vi "MU Load Register.vi"(7 "count in":u32, 8 "error in (no error)":errorcluster, 9 "address":u32, 10 "filepath":string, 11 "handle":u64) -> (0 "error out (no error)":errorcluster, 1 "count out":u32, 2 "values":u32[](array[numeric]), 3 "function return":u32)   [LabVIEW 2017, in "MU_3SL_interface.lvlib"]
uses:
  MU_3SL_interface.lvlib
  lib/MU_3SL_interface.dll
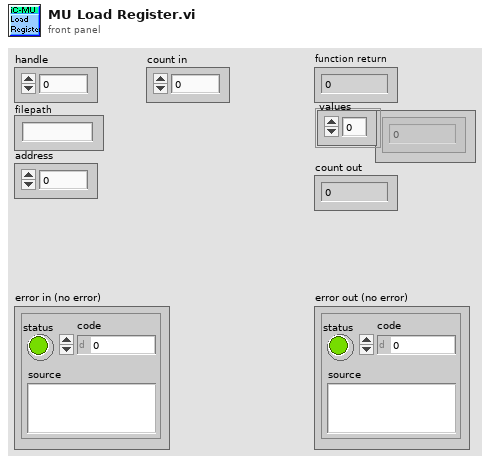
[diagram p1: front panel]
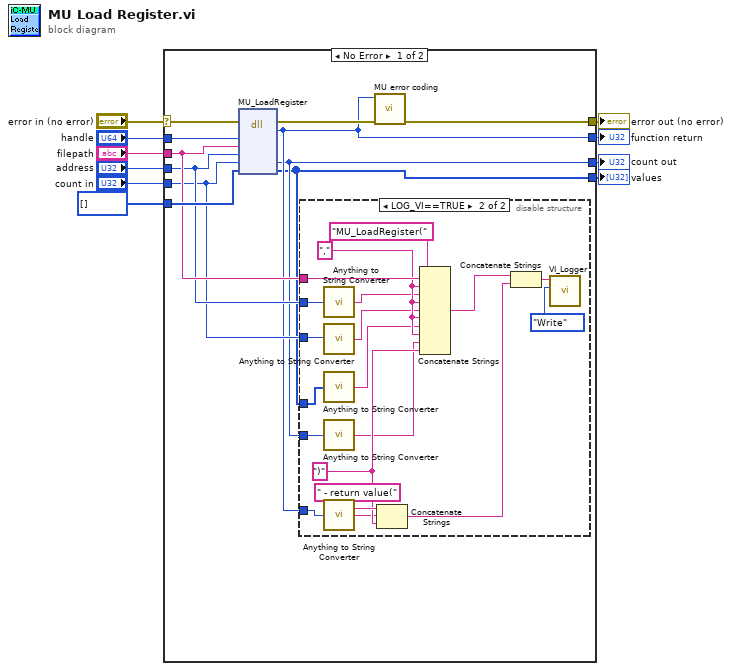
[diagram p0: block diagram]
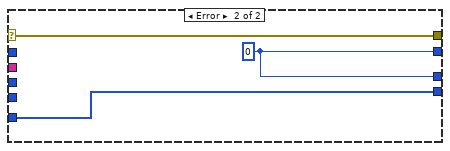
[diagram p3: hidden frame]
diagram:
  n1 = case shown="No Error" "error in (no error)" {
    selector: "error in (no error)" -> [w18 w43]
    tunnel: [w13 w41] -> w10
    tunnel: "handle" -> [w21 _]
    tunnel: "filepath" -> [w16 _]
    tunnel: "address" -> [w15 _]
    tunnel: "count in" -> [w14 _]
    tunnel: [w12 w41] -> w5
    tunnel: [w19 w43] -> w4
    tunnel: [w11 w42] -> w3
    tunnel: u32[] [] ("pulData") -> [w17 w42]
    frame No Error {
      n2 = dll-call lib="C:/Users/bes/AppData/Roaming/work/mu_9so/icsubmodules/soft_mu_3sl_master/lv_interface/lib/MU_3SL_interface**.*" fn="MU_LoadRegister"(error in=w18, "handle"=w21, "filepath"=w16, "address"=w15, "count"=w14, "values"=w17) -> (error out=w20:errorcluster, "return type"=w13:u32, "count"=w12:u32, "values"=w11:u32[])  [unwired: 5 in, 1 out]
      n3 = disable-structure shown="LOG_VI==TRUE" {
        disable-tunnel: w13 -> [_ w23]
        disable-tunnel: w15 -> [_ w32]
        disable-tunnel: w14 -> [_ w30]
        disable-tunnel: w16 -> [_ w35]
        disable-tunnel: w12 -> [_ w25]
        disable-tunnel: w11 -> [_ w28]
        frame condition #0 {
        }
        frame condition #1 (active) {
          w33 = ")" ("string")
          w34 = "," ("string")
          n4 = call "Anything to String Converter.vi"("anything"=w32) -> ("String"=w31:string)
          n5 = call "Anything to String Converter.vi"("anything"=w30) -> ("String"=w29:string)
          n6 = call "Anything to String Converter.vi"("anything"=w28) -> ("String"=w27:string)
          n7 = call "Anything to String Converter.vi"("anything"=w25) -> ("String"=w24:string)
          n8 = call "Anything to String Converter.vi"("anything"=w23) -> ("String"=w22:string)
          n9 = Concatenate Strings(" - return value(" ("string"), w22, w33) -> (w38:string)
          n10 = Concatenate Strings("MU_LoadRegister(" ("Info in"), w35, w34, w31, w34, w29, w34, w27, w34, w24, w33) -> (w26:string)
          n11 = Concatenate Strings(w26, w38) -> (w37:string)
          n12 = call "VI_Logger.vi"("Action (Read)"=enum16{"Write", "Read"}."Write", "Info in"=w37) -> ()  [unwired: 8 in, 2 out]
        }
      }
      n13 = call "MU error coding.vi"("error in (no error)"=w20, "function return in"=w13) -> ("error out"=w19:errorcluster)  [unwired: 9 in]
    }
    frame Error {
      w41 = u32 0 ("return type")
    }
  }
  "function return" <- w10
  "count out" <- w5
  "values" <- w3
  "error out (no error)" <- w4
